vi "Cal_RESTORE.vi"(8 "error in":errorcluster, 10 "Reset ?":bool=TRUE, 11 "VISA name":refnum<visa-resource-name>) -> (0 "error out":errorcluster, 2 "Reset OK ?":bool, 3 "VISA out":refnum<visa-resource-name>)   [LabVIEW 2023, in "QR 10X Eastwood.lvlib"]
uses:
  <instrlib>/QR 10X Eastwood/QR 10X Eastwood.lvlib
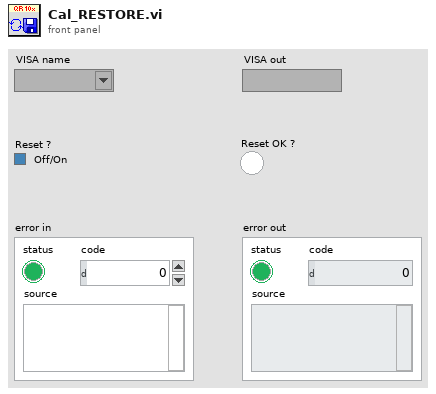
[diagram p1: front panel]
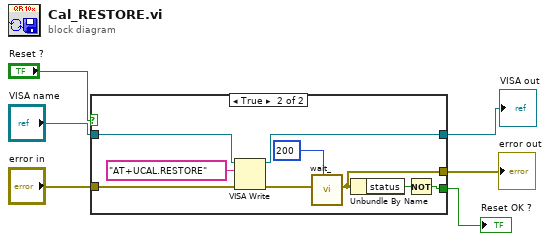
[diagram p0: block diagram]
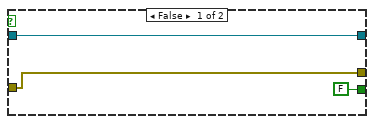
[diagram p2: hidden frame]
diagram:
  n1 = case shown="True" "Reset ?" {
    tunnel: "error in" -> [w8 w17]
    tunnel: "VISA name" -> [w7 w15]
    tunnel: [w8 w11] -> w3
    tunnel: [w7 w18] -> w2
    tunnel: [FALSE w14] -> w1
    frame False {
    }
    frame True {
      n2 = VISA Write(VISA resource name=w15, write buffer="AT+UCAL.RESTORE", error in (no error)=w17) -> (VISA resource name out=w18:refnum<visa-resource-name>, error out=w12:errorcluster)  [unwired: 1 out]
      n3 = call "wait_.vi"("milliseconds to wait"=u32 200, "error in"=w12) -> ("error out"=w11:errorcluster)  [unwired: 9 in]
      n4 = Unbundle By Name(w11) -> ("status"=w13:bool)
      n5 = Not(x=w13) -> (.not. x?=w14:bool)
    }
  }
  "error out" <- w3
  "VISA out" <- w2
  "Reset OK ?" <- w1
